vi "EndGame.vi"(11 "End Game?":bool) -> ()   [LabVIEW 2015]
uses:
  <vilib>/Rock Robotics/WPI/Utilities/WPI_GetSetVariantRefNum.vi
  <vilib>/Rock Robotics/WPI/RobotDrive/WPI_RobotDriveArcadeDrive_Standard(NoSaturation).vi
  <vilib>/Rock Robotics/Network Tables/NT Write Numeric Array.vi
  <vilib>/Rock Robotics/Network Tables/NT Write Number.vi
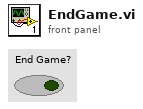
[diagram p1: front panel]
types:
  T1 = typedef "WPI_MotorControlDeviceRef.ctl" = cluster{"DeviceStatus":errorcluster, "Type":T2, "PWM":cluster{"PWM Channel":T3, "DeadBand":T4}, "CAN":cluster{"Device Number":u8, "Control Mode":T5, "Semaphore":T6, "Max Vout":dbl, "TalonSRX Control Mode":T7}, "Invert":bool}
  T2 = typedef "WPI_MotorControlType.ctl" = enum16{"PWM", "CAN", "CANTalonSRX"}
  T3 = typedef "FPGA_DIOPWMChannel.ctl" = enum8{"PWM 0", "PWM 1", "PWM 2", "PWM 3", "PWM 4", "PWM 5", "PWM 6", "PWM 7", "PWM 8", "PWM 9", "PWM MXP 0", "PWM MXP 1", "PWM MXP 2", "PWM MXP 3", "PWM MXP 4", "PWM MXP 5", "PWM MXP 6", "PWM MXP 7", "PWM MXP 8", "PWM MXP 9", "Invalid"}
  T4 = typedef "WPI_PWMDeadband.ctl" = cluster{"Name":string, "maxPositivePwm":i32, "minPositivePwm":i32, "centerPwm":i32, "maxNegativePwm":i32, "minNegativePwm":i32, "angularRange":u16}
  T5 = typedef "WPI_CANJaguar_ControlMode.ctl" = enum8{"Percent VBus", "Current", "Speed", "Position", "Voltage"}
  T6 = typedef "Semaphore RefNum" = refnum<k1>
  T7 = typedef "WPI_CANTalonSRX_APIControlMode.ctl" = enum8{"Percent VBus", "Speed", "Position", "Slave", "Unchanged / Invalid", "Voltage Compensation", "Current", "Motion Profile"}
  T8 = typedef "WPI_RobotDriveDevRef.ctl" = cluster{"DevStatus":errorcluster, "Motors[]":T1[], "Square Inputs":bool, "Max Output":dbl}
  T9 = typedef "WPI_EncoderDevRef.ctl" = cluster{"DevStatus":errorcluster, "EncoderIndex":T10, "CounterIndex":T11, "DistancePerCount":dbl, "Decoding Type":T12}
  T10 = typedef "FPGA_EncoderIdx.ctl" = enum8{"Enc 0", "Enc 1", "Enc 2", "Enc 3", "Enc 4", "Enc 5", "Enc 6", "Enc 7", "Invalid"}
  T11 = typedef "FPGA_CounterCtrSystemIndex.ctl" = enum8{"Ctr 0", "Ctr 1", "Ctr 2", "Ctr 3", "Ctr 4", "Ctr 5", "Ctr 6", "Ctr 7", "Invalid"}
  T12 = typedef "WPI_EncoderType.ctl" = enum16{"1x", "2x", "4x"}
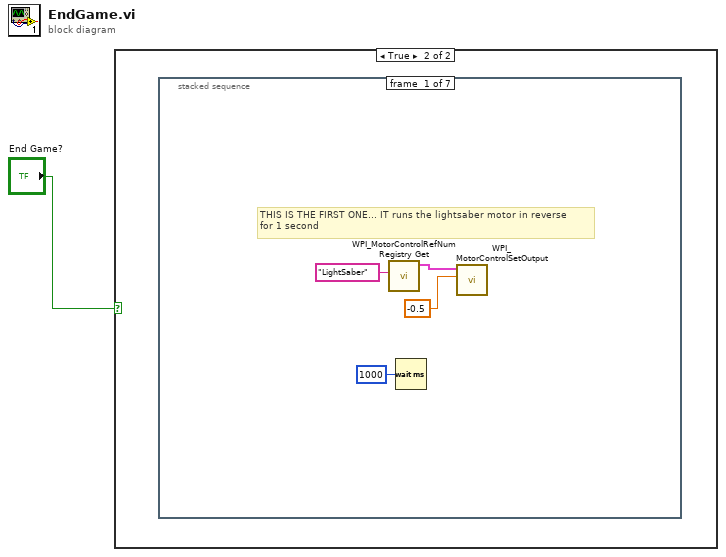
[diagram p0: block diagram]
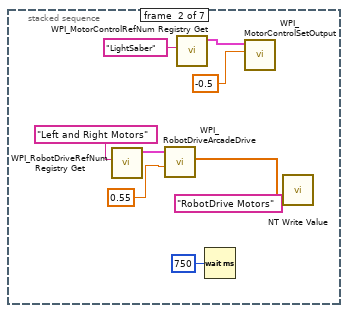
[diagram p3: hidden frame]
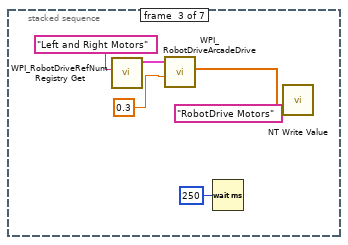
[diagram p4: hidden frame]
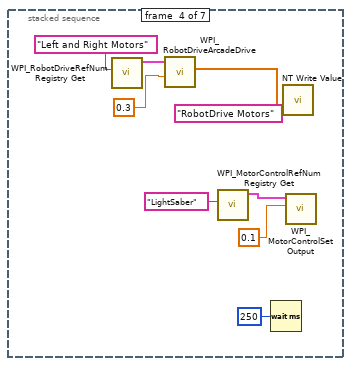
[diagram p5: hidden frame]
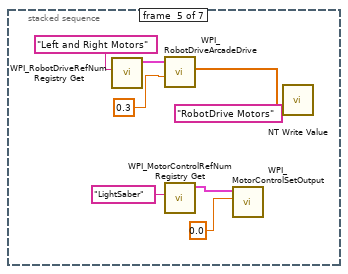
[diagram p6: hidden frame]
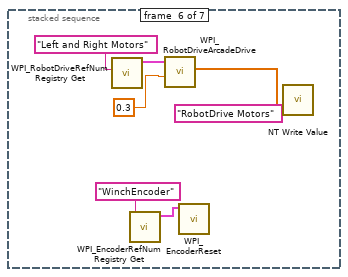
[diagram p7: hidden frame]
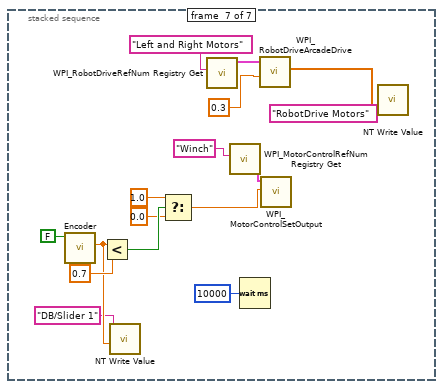
[diagram p8: hidden frame]
diagram:
  n1 = case shown="True" "End Game?" {
    frame False {
    }
    frame True {
      n2 = stacked-sequence {
        frame #0 {
          # "THIS IS THE FIRST ONE... IT runs the lightsaber motor in reverse\nfor 1 second"
          n3 = call <vilib>:"WPI_MotorControlRefNum Registry Get.vi"("refnum name"="LightSaber") -> ("MotorControlDevRef"=w5:T1)  [unwired: 9 in, 1 out]
          n4 = Wait (ms)(milliseconds to wait=u32 1000) -> ()  [unwired: 1 out]
          n5 = call <vilib>:"WPI_MotorControlSetOutput.vi"("Output"=-0.5, "MotorControlDevRef"=w5) -> ()  [unwired: 7 in, 3 out]
        }
        frame #1 {
          n6 = call <vilib>:"WPI_RobotDriveRefNum Registry Get.vi"("refnum name"="Left and Right Motors") -> ("RobotDriveDevRef"=w12:T8)  [unwired: 9 in, 1 out]
          n7 = call-poly <vilib>:"WPI_RobotDriveArcadeDrive.vi"("Y axis value"=0.55 ("X axis value"), "RobotDriveDevRef"=w12) -> ("Motor Values"=w11:dbl[])  [unwired: 7 in, 2 out]
          n8 = call <vilib>:"WPI_MotorControlRefNum Registry Get.vi"("refnum name"="LightSaber") -> ("MotorControlDevRef"=w8:T1)  [unwired: 9 in, 1 out]
          n9 = Wait (ms)(milliseconds to wait=u32 750) -> ()  [unwired: 1 out]
          n10 = call <vilib>:"WPI_MotorControlSetOutput.vi"("Output"=-0.5, "MotorControlDevRef"=w8) -> ()  [unwired: 7 in, 3 out]
          n11 = call-poly <vilib>:"NT Write Value.vi"("Numeric Array"=w11, "Name"="RobotDrive Motors") -> ()  [unwired: 9 in, 1 out]
        }
        frame #2 {
          n12 = call <vilib>:"WPI_RobotDriveRefNum Registry Get.vi"("refnum name"="Left and Right Motors") -> ("RobotDriveDevRef"=w17:T8)  [unwired: 9 in, 1 out]
          n13 = call-poly <vilib>:"WPI_RobotDriveArcadeDrive.vi"("Y axis value"=0.3 ("X axis value"), "RobotDriveDevRef"=w17) -> ("Motor Values"=w16:dbl[])  [unwired: 7 in, 2 out]
          n14 = Wait (ms)(milliseconds to wait=u32 250) -> ()  [unwired: 1 out]
          n15 = call-poly <vilib>:"NT Write Value.vi"("Numeric Array"=w16, "Name"="RobotDrive Motors") -> ()  [unwired: 9 in, 1 out]
        }
        frame #3 {
          n16 = call <vilib>:"WPI_RobotDriveRefNum Registry Get.vi"("refnum name"="Left and Right Motors") -> ("RobotDriveDevRef"=w23:T8)  [unwired: 9 in, 1 out]
          n17 = call-poly <vilib>:"WPI_RobotDriveArcadeDrive.vi"("Y axis value"=0.3 ("X axis value"), "RobotDriveDevRef"=w23) -> ("Motor Values"=w22:dbl[])  [unwired: 7 in, 2 out]
          n18 = call <vilib>:"WPI_MotorControlRefNum Registry Get.vi"("refnum name"="LightSaber") -> ("MotorControlDevRef"=w29:T1)  [unwired: 9 in, 1 out]
          n19 = Wait (ms)(milliseconds to wait=u32 250) -> ()  [unwired: 1 out]
          n20 = call-poly <vilib>:"NT Write Value.vi"("Numeric Array"=w22, "Name"="RobotDrive Motors") -> ()  [unwired: 9 in, 1 out]
          n21 = call <vilib>:"WPI_MotorControlSetOutput.vi"("Output"=0.1, "MotorControlDevRef"=w29) -> ()  [unwired: 7 in, 3 out]
        }
        frame #4 {
          n22 = call <vilib>:"WPI_RobotDriveRefNum Registry Get.vi"("refnum name"="Left and Right Motors") -> ("RobotDriveDevRef"=w32:T8)  [unwired: 9 in, 1 out]
          n23 = call-poly <vilib>:"WPI_RobotDriveArcadeDrive.vi"("Y axis value"=0.3 ("X axis value"), "RobotDriveDevRef"=w32) -> ("Motor Values"=w31:dbl[])  [unwired: 7 in, 2 out]
          n24 = call <vilib>:"WPI_MotorControlRefNum Registry Get.vi"("refnum name"="LightSaber") -> ("MotorControlDevRef"=w35:T1)  [unwired: 9 in, 1 out]
          n25 = call <vilib>:"WPI_MotorControlSetOutput.vi"("Output"=0.0, "MotorControlDevRef"=w35) -> ()  [unwired: 7 in, 3 out]
          n26 = call-poly <vilib>:"NT Write Value.vi"("Numeric Array"=w31, "Name"="RobotDrive Motors") -> ()  [unwired: 9 in, 1 out]
        }
        frame #5 {
          n27 = call <vilib>:"WPI_RobotDriveRefNum Registry Get.vi"("refnum name"="Left and Right Motors") -> ("RobotDriveDevRef"=w40:T8)  [unwired: 9 in, 1 out]
          n28 = call <vilib>:"WPI_EncoderRefNum Registry Get.vi"("refnum name"="WinchEncoder") -> ("EncoderDevRef"=w43:T9)  [unwired: 9 in, 1 out]
          n29 = call-poly <vilib>:"WPI_RobotDriveArcadeDrive.vi"("Y axis value"=0.3 ("X axis value"), "RobotDriveDevRef"=w40) -> ("Motor Values"=w39:dbl[])  [unwired: 7 in, 2 out]
          n30 = call <vilib>:"WPI_EncoderReset.vi"("EncoderDevRef"=w43) -> ()  [unwired: 9 in, 2 out]
          n31 = call-poly <vilib>:"NT Write Value.vi"("Numeric Array"=w39, "Name"="RobotDrive Motors") -> ()  [unwired: 9 in, 1 out]
        }
        frame #6 {
          n32 = call "Encoder.vi"("Reset Encoder?"=FALSE) -> ("revolutions"=w58:dbl)  [unwired: 7 in, 3 out]
          n33 = Less?(x=w58, y=0.7) -> (x < y?=w52:bool)
          n34 = call-poly <vilib>:"NT Write Value.vi"("Numeric"=w58, "Name"="DB/Slider 1") -> ()  [unwired: 9 in, 1 out]
          n35 = Select(t=1.0, s=w52, f=0.0) -> (s? t:f=w53:dbl)
          n36 = call <vilib>:"WPI_RobotDriveRefNum Registry Get.vi"("refnum name"="Left and Right Motors") -> ("RobotDriveDevRef"=w47:T8)  [unwired: 9 in, 1 out]
          n37 = call <vilib>:"WPI_MotorControlRefNum Registry Get.vi"("refnum name"="Winch") -> ("MotorControlDevRef"=w54:T1)  [unwired: 9 in, 1 out]
          n38 = Wait (ms)(milliseconds to wait=u32 10000) -> ()  [unwired: 1 out]
          n39 = call-poly <vilib>:"WPI_RobotDriveArcadeDrive.vi"("Y axis value"=0.3 ("X axis value"), "RobotDriveDevRef"=w47) -> ("Motor Values"=w46:dbl[])  [unwired: 7 in, 2 out]
          n40 = call <vilib>:"WPI_MotorControlSetOutput.vi"("Output"=w53, "MotorControlDevRef"=w54) -> ()  [unwired: 7 in, 3 out]
          n41 = call-poly <vilib>:"NT Write Value.vi"("Numeric Array"=w46, "Name"="RobotDrive Motors") -> ()  [unwired: 9 in, 1 out]
        }
      }
    }
  }
